vi "disconnect.vi"(8 "error in (no error)":errorcluster, 11 "TCPServer in":refnum<class "TCPServer.lvclass">) -> (0 "error out":errorcluster, 3 "TCPServer out":refnum<class "TCPServer.lvclass">)   [LabVIEW 2016, in "TCPServer.lvclass"]
uses:
  TCPServer.lvclass
  C:/Users/aanania/Documents/ts_monochromator_windows/ts_labview_tcp/TCPCommunicator/TCPCommunicator.lvclass
  TCPCommunicator/TCPCommunicator.lvclass/TCPCommunicator.ctl
  TCPCommunicator/TCPCommunicator.lvclass
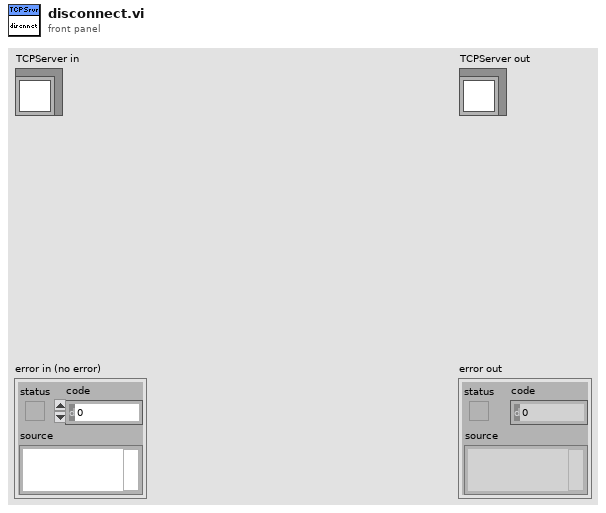
[diagram p1: front panel]
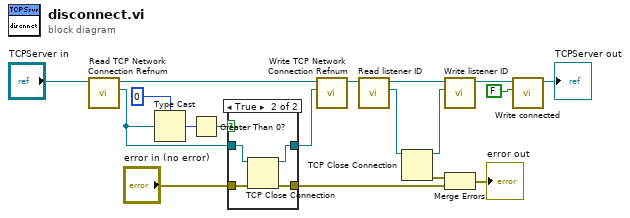
[diagram p0: block diagram]
diagram:
  n1 = call-dynamic "Read TCP Network Connection Refnum.vi"("TCPCommunicator in"="TCPServer in") -> ("TCP Network Connection Refnum"=w4:refnum<k5>, "TCPCommunicator out"=w15:refnum<class "TCPServer.lvclass">)  [unwired: 8 in, 1 out]
  n2 = Type Cast(type=0, x=w4) -> (*(type *) &x=w1:i32)
  n3 = Greater Than 0?(x=w1) -> (x > 0?=w3:bool)
  n4 = case shown="True" w3 {
    tunnel: w4 -> [w19 w24]
    tunnel: "error in (no error)" -> [w20 w23]
    tunnel: [w19 w22] -> w16
    tunnel: [w20 w21] -> w7
    frame False {
    }
    frame True {
      n5 = TCP Close Connection(connection ID=w24, error in (no error)=w23) -> (connection ID out=w22:refnum<k5>, error out=w21:errorcluster)  [unwired: 1 out]
    }
  }
  n6 = call-dynamic "Write TCP Network Connection Refnum.vi"("TCP Network Connection Refnum"=w16, "TCPCommunicator in"=w15) -> ("TCPCommunicator out"=w12:refnum<class "TCPServer.lvclass">)  [unwired: 8 in, 1 out]
  n7 = call "Read listener ID.vi"("TCPCommunicator in"=w12) -> ("listener ID"=w10:refnum<k5>, "TCPCommunicator out"=w11:refnum<class "TCPServer.lvclass">)  [unwired: 8 in, 1 out]
  n8 = TCP Close Connection(connection ID=w10) -> (connection ID out=w9:refnum<k5>, error out=w6:errorcluster)  [unwired: 1 in, 1 out]
  n9 = call "Write listener ID.vi"("listener ID"=w9, "TCPCommunicator in"=w11) -> ("TCPCommunicator out"=w8:refnum<class "TCPServer.lvclass">)  [unwired: 8 in, 1 out]
  n10 = Merge Errors(w6, w7) -> (→"error out":errorcluster)
  n11 = call "Write connected.vi"("connected"=FALSE, "TCPCommunicator in"=w8) -> ("TCPCommunicator out"=→"TCPServer out":refnum<class "TCPServer.lvclass">)  [unwired: 8 in, 1 out]
